vi "Test Self Messaging.vi"() -> ()   [LabVIEW 2020, in "Messaging Tests.lvlib" / "Messaging Tests.lvclass"]
uses:
  Messaging Tests.lvclass
  C:/Program Files/National Instruments/LabVIEW 2024/vi.lib/Astemes/LUnit/Test Case.lvclass
  Core/ActorFramework/LastAck/Last Ack.lvclass
  Self Incrementer/Self Incrementer/Self Incrementer.lvclass
  C:/Users/J63553/Projects/_LabVIEW Community/actor-framework/Core/ActorFramework/Actor/Actor.lvclass
  Core/ActorFramework/Message Queue/Message Queue.lvclass/Message Queue.ctl
  Self Incrementer/Start Increment Msg/Start Increment Msg.lvclass/Start Increment Msg.ctl
  Core/ActorFramework/Message Enqueuer/Message Enqueuer.lvclass/Message Enqueuer.ctl
  Core/ActorFramework/Message Dequeuer/Message Dequeuer.lvclass/Message Dequeuer.ctl
  Core/ActorFramework/LastAck/Last Ack.lvclass/Last Ack.ctl
  Self Incrementer/Self Incrementer/Self Incrementer.lvclass/Self Incrementer.ctl
  <vilib>/Astemes/LUnit/Test Case.lvclass/Test Case.ctl
  6260b4aa-b2d2-4a3b-9cac-94892df10733.vi
  d6fa9793-f178-4552-9720-9b908d0ede32.vi
  <vilib>/Astemes/LUnit/Append Pass Result.vi
  <vilib>/Astemes/LUnit/Append Fail Result.vi
  6260b4aa-b2d2-4a3b-9cac-94892df10733.vi/9c5d11cd-9439-4240-a1ee-d9baace9c924.vi
  d6fa9793-f178-4552-9720-9b908d0ede32.vi/9c5d11cd-9439-4240-a1ee-d9baace9c924.vi
  Core/ActorFramework/Message Enqueuer/Enqueue.vi
  <vilib>/Astemes/LUnit/Run In UI.vi
  <vilib>/Utility/error.llb/Clear Errors.vi
  Self Incrementer/Start Increment Msg/Start Increment Msg.lvclass
  C:/Users/J63553/Projects/_LabVIEW Community/actor-framework/Core/ActorFramework/Message/Message.lvclass
  Core/ActorFramework/Message Priority Queue/Priority Dequeue.vi
  Core/ActorFramework/Message Priority Queue/Priority Enqueue.vi
  Core/ActorFramework/Actor/Actor.lvclass
  Core/ActorFramework/Message Queue/Message Queue.lvclass
  Core/ActorFramework/Message Dequeuer/Message Dequeuer.lvclass
  <vilib>/Astemes/LUnit/Test Case.lvclass
panel:
  out "Test Case Out":refnum<class "Messaging Tests.lvclass">
  in  "Test Case In":refnum<class "Messaging Tests.lvclass">
  out "error out":errorcluster
  in  "error in":errorcluster
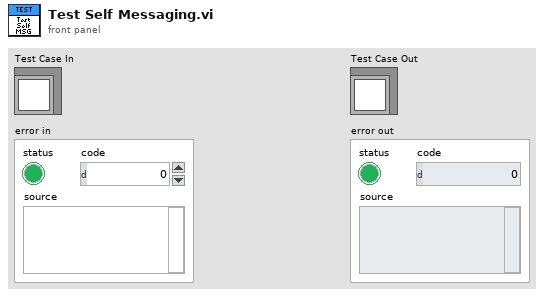
[diagram p1: front panel]
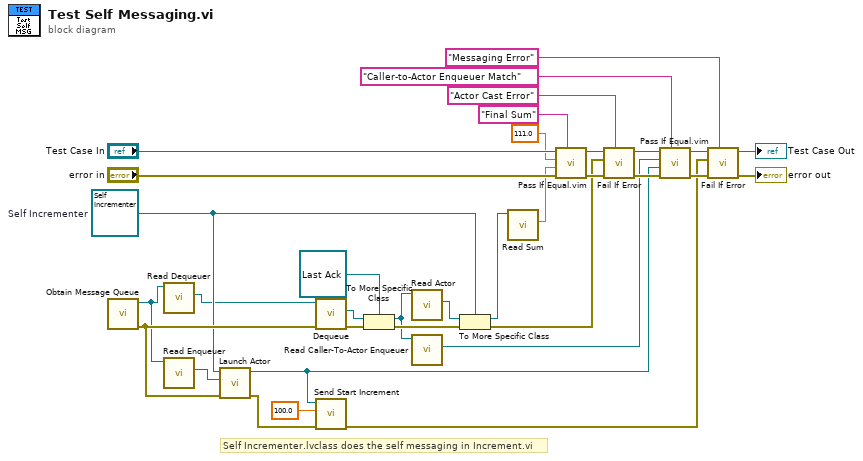
[diagram p0: block diagram]
diagram:
  w2 = refnum<class "Self Incrementer.lvclass"> refnum  # Self Incrementer
  # "Self Incrementer.lvclass does the self messaging in Increment.vi"
  n1 = call "Obtain Message Queue.vi"() -> ("error out"=w24:errorcluster, "Message Queue"=w19:refnum<class "Message Queue.lvclass">)  [unwired: 10 in]
  n2 = call "Read Dequeuer.vi"("Message Queue"=w19) -> ("Message Dequeuer"=w1:refnum<class "Message Dequeuer.lvclass">)  [unwired: 10 in]
  n3 = call "Read Enqueuer.vi"("Message Queue"=w19) -> ("Message Enqueuer"=w18:refnum<class "Message Enqueuer.lvclass">)  [unwired: 10 in]
  n4 = call "Launch Actor.vi"("error in (no error)"=w24, "Actor-to-Caller Enqueuer"=w18, "Actor"=w2) -> ("error out"=w33:errorcluster, "Caller-To-Actor Enqueuer"=w6:refnum<class "Message Enqueuer.lvclass">)  [unwired: 7 in]
  n5 = call "Dequeue.vi"("error in (no error)"=w24, "Message Dequeuer in"=w1) -> ("error out"=w32:errorcluster, "Message"=w17:refnum<class "Message.lvclass">)  [unwired: 5 in, 3 out]
  n6 = call "Send Start Increment.vi"("error in (no error)"=w33, "Numeric"=100.0, "Message Enqueuer"=w6) -> ("error out"=w25:errorcluster)  [unwired: 8 in]
  n7 = To More Specific Class(target class=refnum<class "Last Ack.lvclass"> refnum ("Actor Framework.lvlib:Last Ack"), reference=w17, error in=w32) -> (specific class reference=w16:refnum<class "Last Ack.lvclass">, error out=w34:errorcluster)
  n8 = call "Read Actor.vi"("Last Ack"=w16) -> ("Actor"=w22:refnum<class "Actor.lvclass">)  [unwired: 10 in]
  n9 = call "Read Caller-To-Actor Enqueuer.vi"("Last Ack"=w16) -> ("Caller-to-Actor Enqueuer"=w7:refnum<class "Message Enqueuer.lvclass">)  [unwired: 10 in]
  n10 = To More Specific Class(target class=w2, reference=w22, error in=w34) -> (specific class reference=w20:refnum<class "Self Incrementer.lvclass">, error out=w29:errorcluster)
  n11 = call "Read Sum.vi"("Self Incrementer in"=w20) -> ("Sum"=w12:dbl)  [unwired: 9 in, 1 out]
  n12 = call "Pass If Equal.vim"("Description"="Final Sum", "error in (no error)"="error in", "Actual"=w12, "Expected"=111.0 ("x"), "LUnit Test Case In"="Test Case In") -> ("error out"=w30:errorcluster, "LUnit Test Case Out"=w11:refnum<class "Messaging Tests.lvclass">)  [unwired: 5 in]
  n13 = call <vilib>:"Fail If Error.vi"("Description"="Actor Cast Error", "error in (no error)"=w30, "Assert error"=w29, "LUnit Test Case In"=w11) -> ("error out"=w28:errorcluster, "LUnit Test Case Out"=w9:refnum<class "Messaging Tests.lvclass">)  [unwired: 6 in]
  n14 = call "Pass If Equal.vim"("Description"="Caller-to-Actor Enqueuer Match", "error in (no error)"=w28, "Actual"=w6, "Expected"=w7, "LUnit Test Case In"=w9) -> ("error out"=w27:errorcluster, "LUnit Test Case Out"=w8:refnum<class "Messaging Tests.lvclass">)  [unwired: 5 in]
  n15 = call <vilib>:"Fail If Error.vi"("Description"="Messaging Error", "error in (no error)"=w27, "Assert error"=w25, "LUnit Test Case In"=w8) -> ("error out"=→"error out":errorcluster, "LUnit Test Case Out"=→"Test Case Out":refnum<class "Messaging Tests.lvclass">)  [unwired: 6 in]
